vi "eTdsBLE_ReadData.vi"(0 "eTDS Reference":refnum<k24>, 1 "error in":errorcluster) -> (2 "eTDS Ref Out":refnum<k24>, 3 "BleDataArray":u8[](array[numeric]), 4 "error out":errorcluster)   [LabVIEW 2013]
uses:
  D:/GitHub/GT-Bionics/TDS-HM/Labview Code/C# BLE Interface/eTDS BLE Interface/TdsBleInterface for LV/TdsForLV/TdsForLV/bin/TdsForLV.dll
  TdsForLV/TdsForLV/bin/TdsForLV.dll
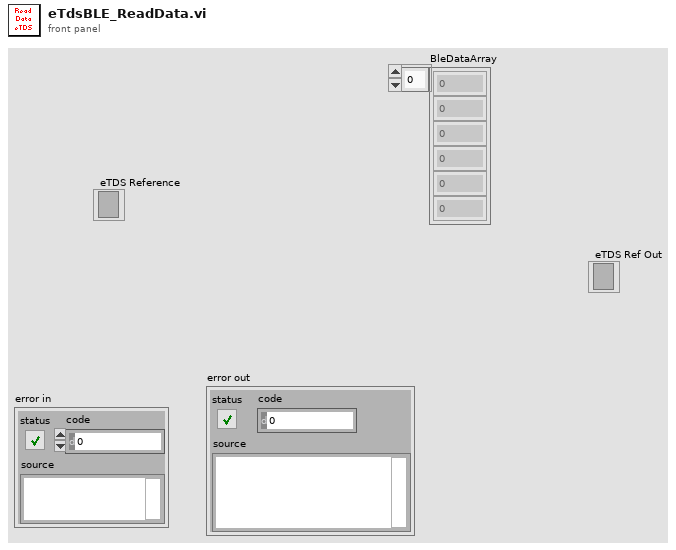
[diagram p1: front panel]
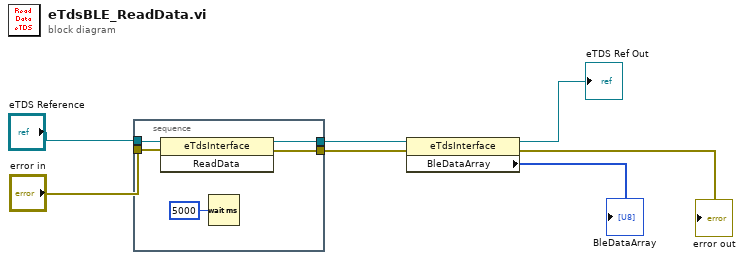
[diagram p0: block diagram]
diagram:
  n1 = stacked-sequence {
    tunnel: "eTDS Reference" -> [w12]
    tunnel: "error in" -> [w11]
    tunnel: [w10] -> w6
    tunnel: [w9] -> w5
    frame #0 {
      n2 = invoke class="eTdsInterface" method="ReadData"(reference=w12, error in=w11) -> (reference out=w10:refnum<k24>, error out=w9:errorcluster)  [unwired: 1 in, 1 out]
      n3 = Wait (ms)(milliseconds to wait=u32 5000) -> ()  [unwired: 1 out]
    }
  }
  n4 = property class="eTdsInterface"(reference=w6, error in=w5) -> (reference out=→"eTDS Ref Out":refnum<k24>, error out=→"error out":errorcluster, "BleDataArray"=→"BleDataArray":u8[])
